vi "Teleop.vi"(10 "Match Info":T1={"Autonomous Elapsed Seconds"=0.0, "TeleOp Elapsed Seconds"=0.0, "Disabled Elapsed Seconds"=0.0, "Visited Autonomous"=FALSE, "Visited TeleOp"=FALSE, "Visited Disabled"=FALSE, "Autonomous Settings"={"Autonomous Style"=enum."Independent", "VI Refnum"=refnum}}, 11 "Call Context":T2) -> ()   [LabVIEW 2017]
doc: "This VI is called for each TeleOp packet received from the DS where the robot is not disabled. It is often used to read from the joysticks and update I/O or to update setpoints for timed control loops. It should complete and return within 20 milliseconds or it may miss DS packets."
uses:
  <vilib>/Rock Robotics/WPI/DriverStation/WPI_DriverStationDerivedRobotMode.ctl
  <vilib>/Rock Robotics/WPI/DriverStation/WPI_DriverStationMatch Info.ctl
  <vilib>/Rock Robotics/WPI/Solenoid/WPI_SolenoidValue.ctl
  Change Detect.vi
  Change Detect Boolean.vi
  <vilib>/Rock Robotics/WPI/Utilities/WPI_GetSetVariantRefNum.vi
  <vilib>/Rock Robotics/WPI/Solenoid/WPI_SolenoidSetEnum.vi
panel:
  out "Boolean":bool
  in  "constante":dbl=0.3 format="%#_13g"
  in  "puxa":dbl=0.6 format="%#_13g"
  in  "expele":dbl=-0.6 format="%#_13g"
  in  "negInertiaScalar":dbl=0.8
  in  "Sensitivty":dbl=1.15
  in  "WheelNonLinearity":dbl=0.65
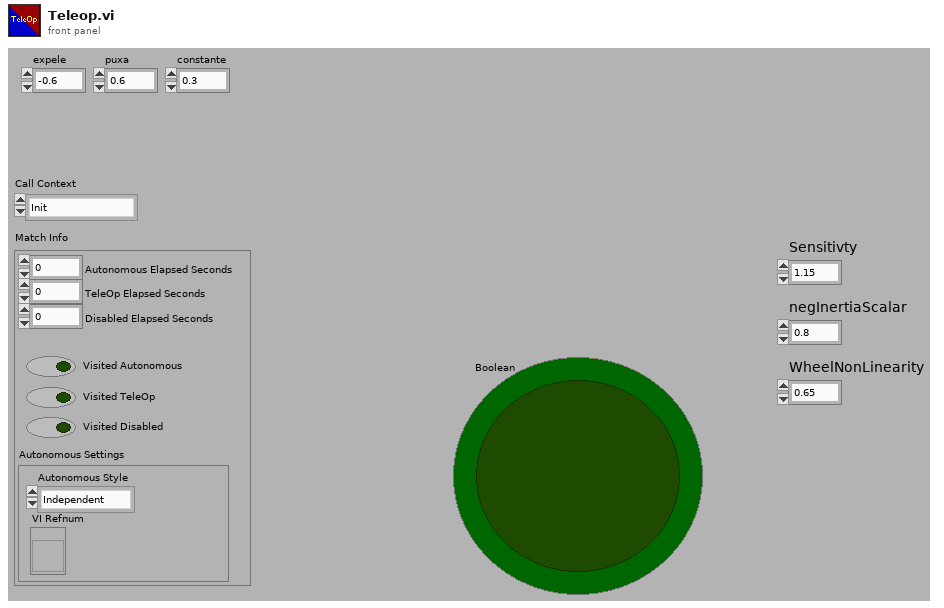
[diagram p1: front panel]
types:
  T1 = typedef "WPI_DriverStationMatch Info.ctl" = cluster{"Autonomous Elapsed Seconds":dbl, "TeleOp Elapsed Seconds":dbl, "Disabled Elapsed Seconds":dbl, "Visited Autonomous":bool, "Visited TeleOp":bool, "Visited Disabled":bool, "Autonomous Settings":cluster{"Autonomous Style":enum16{"Iterative", "Independent"}, "VI Refnum":refnum<vi>}}
  T2 = typedef "WPI_DriverStationDerivedRobotMode.ctl" = enum16{"Init", "Execute", "Stop"}
  T3 = typedef "WPI_SolenoidValue.ctl" = enum16{"Off", "On", "Forward", "Reverse"}
  T4 = typedef "WPI_JoystickDevRef.ctl" = cluster{"Device":T5}
  T5 = typedef "WPI_JoystickDeviceEnum.ctl" = enum16{"USB 0", "USB 1", "USB 2", "USB 3", "USB 4", "USB 5"}
  T6 = cluster{"Buttons[0]":bool, "Buttons[1]":bool, "Buttons[2]":bool, "Buttons[3]":bool, "Buttons[4]":bool, "Buttons[5]":bool, "Buttons[6]":bool, "Buttons[7]":bool, "Buttons[8]":bool}
  T7 = typedef "WPI_SwitchDevRef.ctl" = cluster{"DevStatus":errorcluster, "DIO Channel":T8, "CntIndex":T9, "Normally Closed":bool}
  T8 = typedef "FPGA_DIOChannel.ctl" = enum8{"DIO 0", "DIO 1", "DIO 2", "DIO 3", "DIO 4", "DIO 5", "DIO 6", "DIO 7", "DIO 8", "DIO 9", "DIO MXP 0", "DIO MXP 1", "DIO MXP 2", "DIO MXP 3", "DIO MXP 4", "DIO MXP 5", "DIO MXP 6", "DIO MXP 7", "DIO MXP 8", "DIO MXP 9", "DIO MXP 10", "DIO MXP 11", "DIO MXP 12", "DIO MXP 13", "DIO MXP 14", "DIO MXP 15", "SPI Port CS1", "SPI Port CS2", "SPI Port CS3", "SPI Port MISO", "SPI Port MOSI", "Invalid"}
  T9 = typedef "FPGA_CounterCtrSystemIndex.ctl" = enum8{"Ctr 0", "Ctr 1", "Ctr 2", "Ctr 3", "Ctr 4", "Ctr 5", "Ctr 6", "Ctr 7", "Invalid"}
  T10 = typedef "WPI_MotorControlDeviceRef.ctl" = cluster{"DeviceStatus":errorcluster, "Type":T11, "PWM":cluster{"PWM Channel":T12, "DeadBand":T13}, "CAN":cluster{"Device Number":u8, "SetOutput VI Ref":variant, "GetOutput VI Ref":variant, "Enable VI Ref":variant, "Disable VI Ref":variant, "Data":variant}, "Invert":bool, "DIO PWM":cluster{"PWM \"Enable\" Channel":T12, "DIOChannel":T8, "PWM Rate":dbl}}
  T11 = typedef "WPI_MotorControlType.ctl" = enum16{"PWM", "CAN", "DIO PWM"}
  T12 = typedef "FPGA_DIOPWMChannel.ctl" = enum8{"PWM 0", "PWM 1", "PWM 2", "PWM 3", "PWM 4", "PWM 5", "PWM 6", "PWM 7", "PWM 8", "PWM 9", "PWM MXP 0", "PWM MXP 1", "PWM MXP 2", "PWM MXP 3", "PWM MXP 4", "PWM MXP 5", "PWM MXP 6", "PWM MXP 7", "PWM MXP 8", "PWM MXP 9", "Invalid"}
  T13 = typedef "WPI_PWMDeadband.ctl" = cluster{"Name":string, "maxPositivePwm":i32, "minPositivePwm":i32, "centerPwm":i32, "maxNegativePwm":i32, "minNegativePwm":i32, "angularRange":u16}
  T14 = typedef "WPI_RobotDriveDevRef.ctl" = cluster{"DevStatus":errorcluster, "Motors[]":T10[], "Square Inputs":bool, "Max Output":dbl}
  T15 = cluster{"Axes[0]":dbl, "Axes[1]":dbl, "Axes[2]":dbl, "Axes[3]":dbl, "Axes[4]":dbl, "Axes[5]":dbl, "Axes[6]":dbl, "Axes[7]":dbl, "Axes[8]":dbl}
  T16 = typedef "WPI_SolenoidDevRef.ctl" = cluster{"DevStatus":errorcluster, "Pneumatics Control Module":u8, "Forward Solenoid Channel":T17, "Reverse Solenoid Channel":T17}
  T17 = typedef "WPI_SolenoidChannel.ctl" = enum8{"Solenoid 0", "Solenoid 1", "Solenoid 2", "Solenoid 3", "Solenoid 4", "Solenoid 5", "Solenoid 6", "Solenoid 7", "Invalid"}
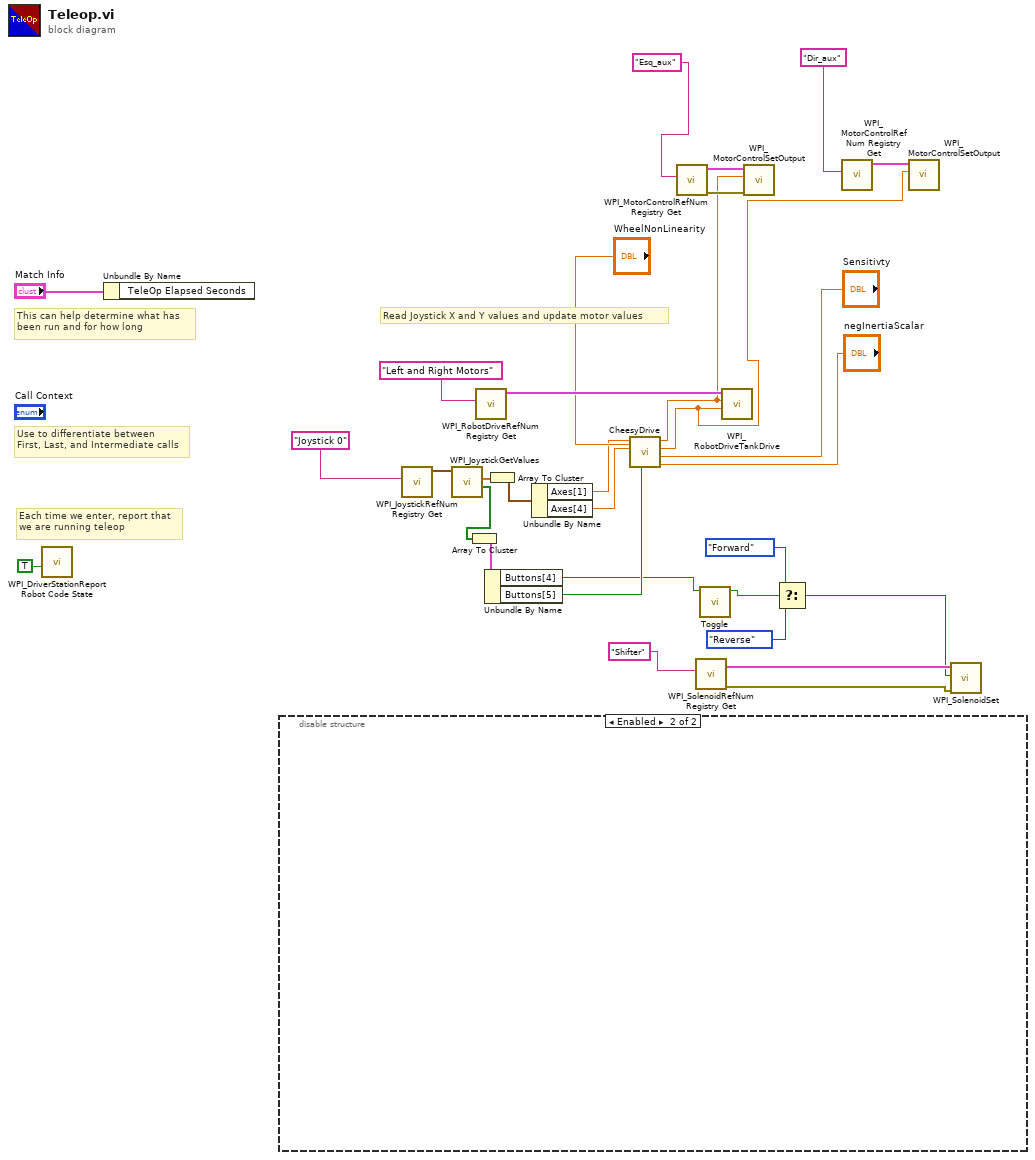
[diagram p0: block diagram]
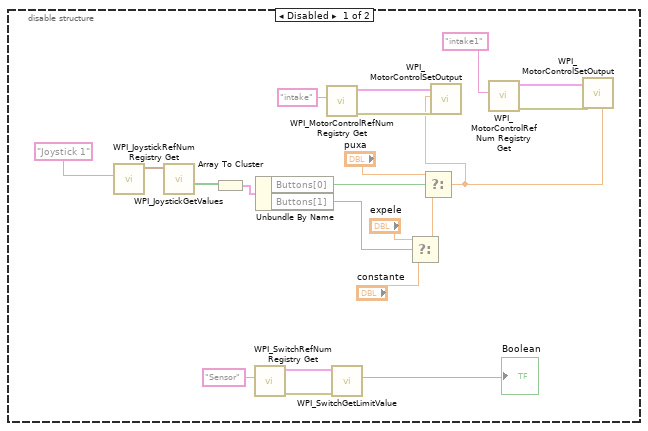
[diagram p2: hidden frame]
diagram:
  # "Each time we enter, report that\nwe are running teleop"
  # "Use to differentiate between\nFirst, Last, and Intermediate calls"
  # "This can help determine what has\nbeen run and for how long"
  # "Read Joystick X and Y values and update motor values"
  n1 = call <vilib>:"WPI_DriverStationReport Robot Code State.vi"("TeleOp"=TRUE ("Autonomous")) -> ()  [unwired: 10 in, 1 out]
  n2 = Unbundle By Name("Match Info") -> ()  [unwired: 1 out]
  n3 = disable-structure shown="Enabled" {
    frame Disabled {
      n4 = call <vilib>:"WPI_JoystickRefNum Registry Get.vi"("refnum name"="Joystick 1") -> ("JoystickDevRef"=w49:T4)  [unwired: 1 in, 9 out]
      n5 = call <vilib>:"WPI_JoystickGetValues.vi"("JoystickDevRef"=w49) -> ("Buttons"=w48:bool[])  [unwired: 6 in, 4 out]
      n6 = Array To Cluster(array=w48) -> (cluster=w47:T6)
      n7 = call <vilib>:"WPI_SwitchRefNum Registry Get.vi"("refnum name"="Sensor") -> ("error out"=w35:errorcluster, "SwitchDevRef"=w36:T7)  [unwired: 9 in]
      n8 = Unbundle By Name(w47) -> ("Buttons[0]"=w32:bool, "Buttons[1]"=w45:bool)
      n9 = call <vilib>:"WPI_MotorControlRefNum Registry Get.vi"("refnum name"="intake") -> ("error out"=w51:errorcluster, "MotorControlDevRef"=w52:T10)  [unwired: 9 in]
      n10 = call <vilib>:"WPI_SwitchGetLimitValue.vi"("error in (no error)"=w35, "SwitchDevRef"=w36) -> ("Switch Pressed"=→"Boolean":bool)  [unwired: 7 in, 2 out]
      n11 = Select(t="expele", s=w45, f="constante") -> (s? t:f=w43:dbl)
      n12 = Select(t="puxa", s=w32, f=w43) -> (s? t:f=w38:dbl)
      n13 = call <vilib>:"WPI_MotorControlSetOutput.vi"("error in (no error)"=w51, "Output"=w38, "MotorControlDevRef"=w52) -> ()  [unwired: 6 in, 3 out]
      n14 = call <vilib>:"WPI_MotorControlRefNum Registry Get.vi"("refnum name"="intake1") -> ("error out"=w41:errorcluster, "MotorControlDevRef"=w37:T10)  [unwired: 9 in]
      n15 = call <vilib>:"WPI_MotorControlSetOutput.vi"("error in (no error)"=w41, "Output"=w38, "MotorControlDevRef"=w37) -> ()  [unwired: 6 in, 3 out]
    }
    frame Enabled {
    }
  }
  n16 = call <vilib>:"WPI_JoystickRefNum Registry Get.vi"("refnum name"="Joystick 0") -> ("JoystickDevRef"=w27:T4)  [unwired: 1 in, 9 out]
  n17 = call <vilib>:"WPI_JoystickGetValues.vi"("JoystickDevRef"=w27) -> ("Buttons"=w21:bool[], "Axes"=w25:dbl[])  [unwired: 6 in, 3 out]
  n18 = Array To Cluster(array=w21) -> (cluster=w22:T6)
  n19 = call <vilib>:"WPI_RobotDriveRefNum Registry Get.vi"("refnum name"="Left and Right Motors") -> ("RobotDriveDevRef"=w29:T14)  [unwired: 1 in, 9 out]
  n20 = Unbundle By Name(w22) -> ("Buttons[4]"=w8:bool, "Buttons[5]"=w10:bool)
  n21 = Array To Cluster(array=w25) -> (cluster=w24:T15)
  n22 = Unbundle By Name(w24) -> ("Axes[1]"=w20:dbl, "Axes[4]"=w19:dbl)
  n23 = call "CheesyDrive.vi"("Quickturn"=w10, "WheelNonLinearity"="WheelNonLinearity", "negInertiaScalar"="negInertiaScalar", "Sensitivty"="Sensitivty", "Wheel"=w19, "Throttle"=w20) -> ("Right PWM"=w1:dbl, "Left PWM"=w4:dbl)  [unwired: 4 in]
  n24 = call <vilib>:"WPI_MotorControlRefNum Registry Get.vi"("refnum name"="Esq_aux") -> ("error out"=w6:errorcluster, "MotorControlDevRef"=w7:T10)  [unwired: 9 in]
  n25 = call <vilib>:"WPI_SolenoidRefNum Registry Get.vi"("refnum name"="Shifter") -> ("error out"=w14:errorcluster, "SolenoidDevRef"=w15:T16)  [unwired: 9 in]
  n26 = call "Toggle.vi"("In"=w8) -> ("Toggled"=w9:bool)  [unwired: 10 in]
  n27 = call <vilib>:"WPI_RobotDriveTankDrive.vi"("Right axis value"=w1, "Left axis value"=w4, "RobotDriveDevRef"=w29) -> ()  [unwired: 6 in, 3 out]
  n28 = call <vilib>:"WPI_MotorControlSetOutput.vi"("error in (no error)"=w6, "Output"=w4, "MotorControlDevRef"=w7) -> ()  [unwired: 6 in, 3 out]
  n29 = Select(t=WPI_SolenoidValue."Forward" ("Value"), s=w9, f=WPI_SolenoidValue."Reverse" ("Value")) -> (s? t:f=w11:T3)
  n30 = call <vilib>:"WPI_MotorControlRefNum Registry Get.vi"("refnum name"="Dir_aux") -> ("MotorControlDevRef"=w3:T10)  [unwired: 9 in, 1 out]
  n31 = call <vilib>:"WPI_MotorControlSetOutput.vi"("Output"=w1, "MotorControlDevRef"=w3) -> ()  [unwired: 7 in, 3 out]
  n32 = call-poly <vilib>:"WPI_SolenoidSet.vi"("error in (no error)"=w14, "Value"=w11, "SolenoidDevRef"=w15) -> ()  [unwired: 7 in, 2 out]
